vi "Waveform preset.vi"(11 "Galvo signal":u32) -> ()   [LabVIEW 2015]
uses:
  <vilib>/rvi/eio/common/nirviEmuTemplateMethod_errors.vi
  <vilib>/eio/EIONode/EIONode.xnode
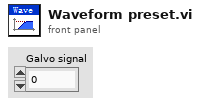
[diagram p1: front panel]
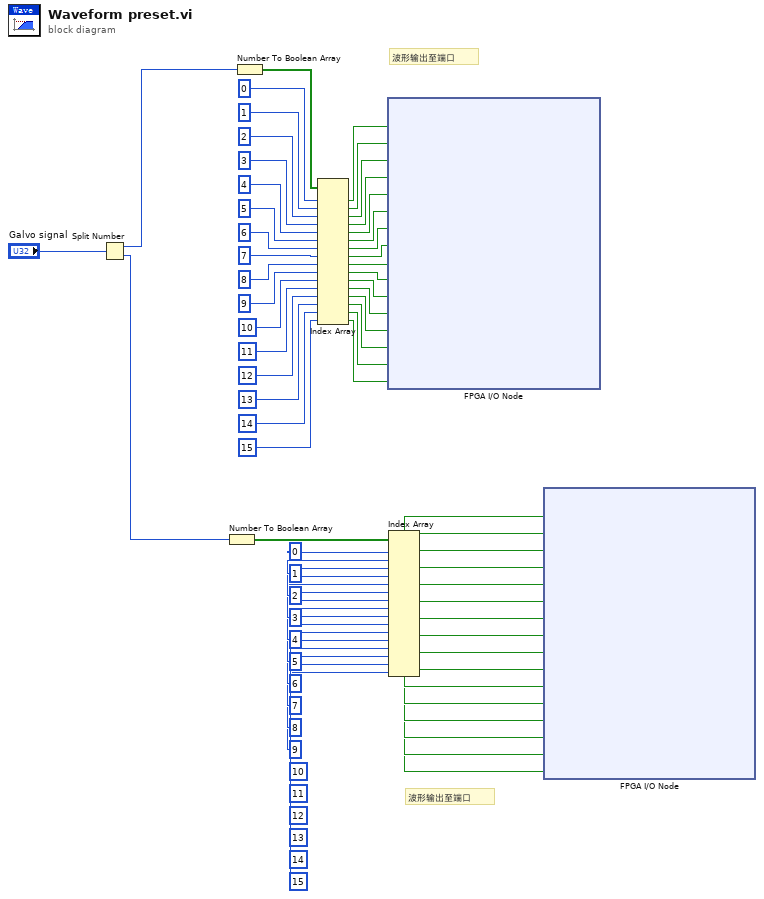
[diagram p0: block diagram]
diagram:
  # "波形输出至端口"
  # "波形输出至端口"
  n1 = Split Number(x="Galvo signal") -> (hi(x)=w2:u16, lo(x)=w1:u16)
  n2 = Number To Boolean Array(number=w1) -> (Boolean array=w3:bool[])
  n3 = Number To Boolean Array(number=w2) -> (Boolean array=w68:bool[])
  n4 = Index Array(array=w68, index #1=0 ("index"), index #2=1 ("index"), index #3=2 ("index"), index #4=3 ("index"), index #5=4 ("index"), index #6=5 ("index"), index #7=6 ("index"), index #8=7 ("index"), index #9=8 ("index"), index #10=9 ("index"), index #11=10 ("index"), index #12=11 ("index"), index #13=12 ("index"), index #14=13 ("index"), index #15=14 ("index"), index #16=15 ("index")) -> (element #1=w51:bool, element #2=w50:bool, element #3=w49:bool, element #4=w48:bool, element #5=w47:bool, element #6=w46:bool, element #7=w45:bool, element #8=w44:bool, element #9=w43:bool, element #10=w42:bool, element #11=w41:bool, element #12=w40:bool, element #13=w39:bool, element #14=w38:bool, element #15=w37:bool, element #16=w36:bool)
  n5 = xnode "FPGA I/O Node"("IO Module\\DDCA_DIO8_WRITE"=w51, "IO Module\\DDCA_DIO9_WRITE"=w50, "IO Module\\DDCA_DIO10_WRITE"=w49, "IO Module\\DDCA_DIO11_WRITE"=w48, "IO Module\\DDCA_DIO12_WRITE"=w47, "IO Module\\DDCA_DIO13_WRITE"=w46, "IO Module\\DDCA_DIO14_WRITE"=w45, "IO Module\\DDCA_DIO15_WRITE"=w44, "IO Module\\DDCA_DIO16_WRITE"=w43, "IO Module\\DDCA_DIO17_WRITE"=w42, "IO Module\\DDCA_DIO18_WRITE"=w41, "IO Module\\DDCA_DIO19_WRITE"=w40, "IO Module\\DDCA_DIO20_WRITE"=w39, "IO Module\\DDCA_DIO21_WRITE"=w38, "IO Module\\DDCA_DIO22_WRITE"=w37, "IO Module\\DDCA_DIO23_WRITE"=w36) -> ()  [unwired: 16 in, 16 out]
  n6 = Index Array(array=w3, index #1=0 ("index"), index #2=1 ("index"), index #3=2 ("index"), index #4=3 ("index"), index #5=4 ("index"), index #6=5 ("index"), index #7=6 ("index"), index #8=7 ("index"), index #9=8 ("index"), index #10=9 ("index"), index #11=10 ("index"), index #12=11 ("index"), index #13=12 ("index"), index #14=13 ("index"), index #15=14 ("index"), index #16=15 ("index")) -> (element #1=w19:bool, element #2=w18:bool, element #3=w17:bool, element #4=w16:bool, element #5=w15:bool, element #6=w14:bool, element #7=w13:bool, element #8=w12:bool, element #9=w11:bool, element #10=w10:bool, element #11=w9:bool, element #12=w8:bool, element #13=w7:bool, element #14=w6:bool, element #15=w5:bool, element #16=w4:bool)
  n7 = xnode "FPGA I/O Node"("IO Module\\DDCB_DIO8_WRITE"=w19, "IO Module\\DDCB_DIO9_WRITE"=w18, "IO Module\\DDCB_DIO10_WRITE"=w17, "IO Module\\DDCB_DIO11_WRITE"=w16, "IO Module\\DDCB_DIO12_WRITE"=w15, "IO Module\\DDCB_DIO13_WRITE"=w14, "IO Module\\DDCB_DIO14_WRITE"=w13, "IO Module\\DDCB_DIO15_WRITE"=w12, "IO Module\\DDCB_DIO16_WRITE"=w11, "IO Module\\DDCB_DIO17_WRITE"=w10, "IO Module\\DDCB_DIO18_WRITE"=w9, "IO Module\\DDCB_DIO19_WRITE"=w8, "IO Module\\DDCB_DIO20_WRITE"=w7, "IO Module\\DDCB_DIO21_WRITE"=w6, "IO Module\\DDCB_DIO22_WRITE"=w5, "IO Module\\DDCB_DIO23_WRITE"=w4) -> ()  [unwired: 16 in, 16 out]
